vi "ESTOP.vi"(7 "Get/Set":enum16{"Get", "Set"}(ring), 10 "Value In":bool) -> (2 "Value Out":bool)   [LabVIEW 2017]
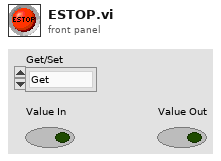
[diagram p1: front panel]
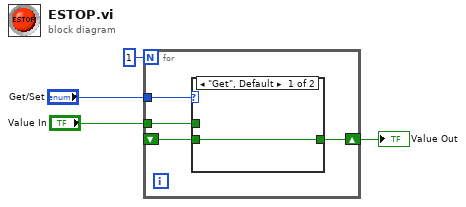
[diagram p0: block diagram]
diagram:
  n1 = for {
    N: 1 -> [_]
    tunnel: "Get/Set" -> [w8]
    tunnel: "Value In" -> [w7]
    shift-right: [w6] -> w1
    shift-left: _ -> [w5]
    n2 = case shown="\"Get\", Default" w8 {
      tunnel: w7 -> [_ w10]
      tunnel: [w9 w10] -> w6
      tunnel: w5 -> [w9 _]
      frame "Get", Default {
      }
      frame "Set" {
      }
    }
  }
  "Value Out" <- w1
